vi "_phase_correction_(Phase_correction).vi"(4 "offset":dbl, 5 "Delay (ns)":dbl, 7 "f1 (GHz)":dbl, 8 "f0 (GHz)":dbl, 9 "Phase in":dbl[](array[numeric])) -> (3 "Phase out":dbl[](array[numeric]))   [LabVIEW 2013]
panel:
  out "Waveform Graph 2":dbl[](graph)
  out "Waveform Graph":dbl[](graph)
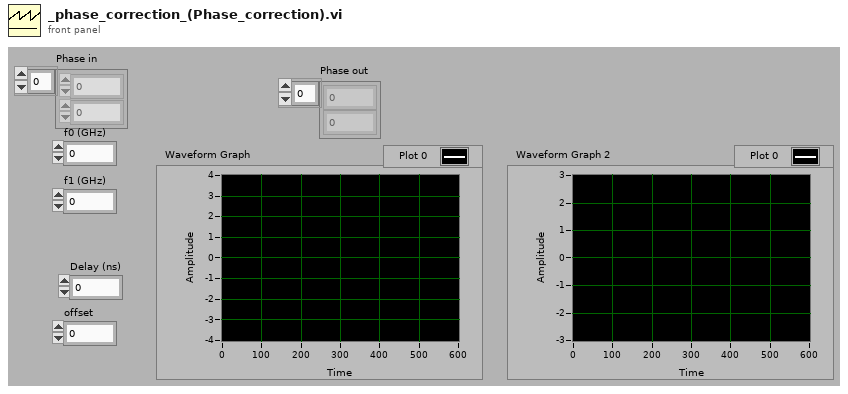
[diagram p1: front panel]
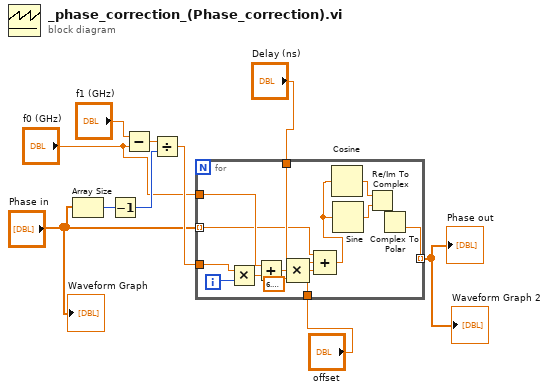
[diagram p0: block diagram]
diagram:
  n1 = Array Size(array="Phase in") -> (size(s)=w10:i32)
  n2 = Decrement(x=w10) -> (x-1=w8:i32)
  n3 = Subtract(x="f1 (GHz)", y="f0 (GHz)") -> (x-y=w9:dbl)
  n4 = Divide(x=w9, y=w8) -> (x/y=w7:dbl)
  n5 = for {
    tunnel: w7 -> [w24]
    tunnel: "f0 (GHz)" -> [w22]
    tunnel: "Delay (ns)" -> [w20]
    tunnel: "Phase in" -> [w18] mode=indexing
    tunnel: [w12] -> w1 mode=indexing
    tunnel: "offset" -> [w11]
    i -> [w25]
    n6 = Multiply(x=w24, y=w25) -> (x*y=w23:dbl)
    n7 = Add(x=w22, y=w23) -> (x+y=w21:dbl)
    n8 = Compound Arithmetic op=MULTIPLY(w20, w21, 6.283185307179586) -> (w19:dbl)
    n9 = Compound Arithmetic op=ADD(w18, w19, w11) -> (w16:dbl)
    n10 = Cosine(x=w16) -> (cos(x)=w14:dbl)
    n11 = Sine(x=w16) -> (sin(x)=w15:dbl)
    n12 = Re/Im To Complex(1:w15, 2:w14) -> (0:w13:cdb)
    n13 = Complex To Polar(r * e^(i*theta)=w13) -> (theta=w12:dbl)  [unwired: 1 out]
  }
  "Phase out" <- w1
  "Waveform Graph 2" <- w1
  "Waveform Graph" <- "Phase in"
